vi "Digit fixed number.vi"(10 "Digit/character number":dbl, 11 "Input":string) -> (3 "Output":string)   [LabVIEW 2020]
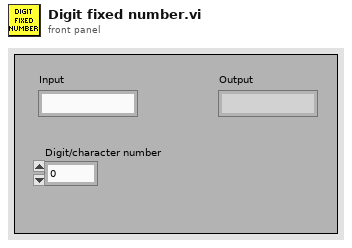
[diagram p1: front panel]
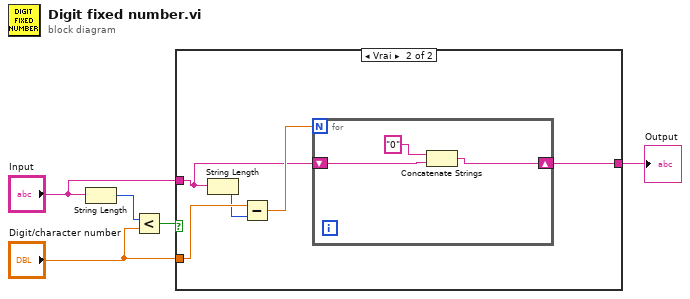
[diagram p0: block diagram]
diagram:
  n1 = String Length(string="Input") -> (length=w5:i32)
  n2 = Less?(x=w5, y="Digit/character number") -> (x < y?=w4:bool)
  n3 = case shown="Vrai" w4 {
    tunnel: "Input" -> [w6 w10]
    tunnel: "Digit/character number" -> [_ w8]
    tunnel: [w6 w9] -> w1
    frame False {
    }
    frame True {
      n4 = String Length(string=w10) -> (length=w7:i32)
      n5 = Subtract(x=w8, y=w7) -> (x-y=w11:dbl)
      n6 = for {
        N: w11 -> [_]
        shift-right: [w13] -> w9
        shift-left: w10 -> [w14]
        n7 = Concatenate Strings("0", w14) -> (w13:string)
      }
    }
  }
  "Output" <- w1
